vi "Find Nearest Power of Ten.vi"(11 "n":dbl) -> (3 "nearest power of ten":dbl)   [LabVIEW 2017, in "NI_Robotics_Configure Steering Frame.lvlib"]
uses:
  <vilib>/robotics/Dialog/Configure Steering Frame/NI_Robotics_Configure Steering Frame.lvlib
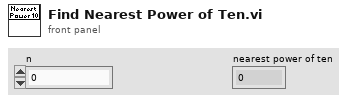
[diagram p1: front panel]
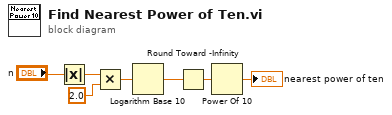
[diagram p0: block diagram]
diagram:
  n1 = Absolute Value(x="n") -> (abs(x)=w6:dbl)
  n2 = Multiply(x=w6, y=2.0) -> (x*y=w4:dbl)
  n3 = Logarithm Base 10(1:w4) -> (0:w3:dbl)
  n4 = Round Toward -Infinity(1:w3) -> (0:w2:dbl)
  n5 = Power Of 10(x=w2) -> (10^x=→"nearest power of ten":dbl)
